vi "Set Live img window UI from file-DBL.vi"(8 "error in (no error)":errorcluster, 9 "Keys setup.DBL":T2, 10 "Section name":string, 11 "Refnum in":T1) -> (0 "error out":errorcluster, 3 "Refnum out":T1)   [LabVIEW 2020]
uses:
  Typedefs/Ini file interface (DBL).ctl
  <vilib>/Utility/config.llb/Config Data RefNum.ctl
  User Interface/Globals/gl_Windows Ctrl refs.vi
  <vilib>/Utility/config.llb/NI_LVConfig.lvlib
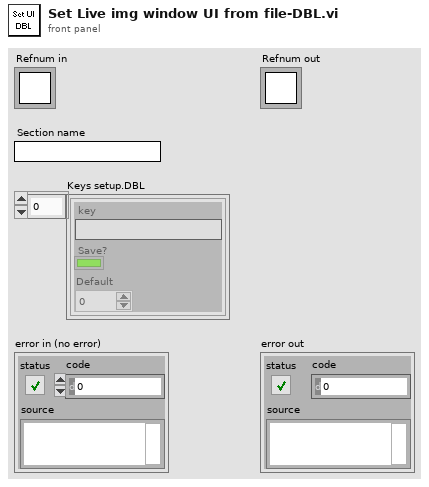
[diagram p1: front panel]
types:
  T1 = typedef "NI_LVConfig.lvlib/Config Data RefNum.ctl" = refnum<k1>
  T2 = typedef "Ini file interface (DBL).ctl" = cluster{"key":string, "Save?":bool, "Default":dbl}[]
  T3 = typedef "Live window-ctrl refs.ctl" = cluster{"This VI":refnum<vi>, "Pane":refnum<vi>, "Show REF Image Left":refnum<vi>, "Show REF Image Right":refnum<vi>, "Snapshot":refnum<vi>, "Left Image Palette":refnum<vi>, "Right Image Palette":refnum<vi>, "Left Channel":refnum<vi>, "Right Channel":refnum<vi>, "Left image intensity":refnum<vi>, "Right image intensity":refnum<vi>, "Left Image Display":T4, "Right Image Display":T4, "Refresh rate ind (Hz)":refnum<vi>, "Acq rate ind (Hz)":refnum<vi>, "Stop (ind)":refnum<vi>}
  T4 = typedef "Image display ref.ctl" = refnum<vi>
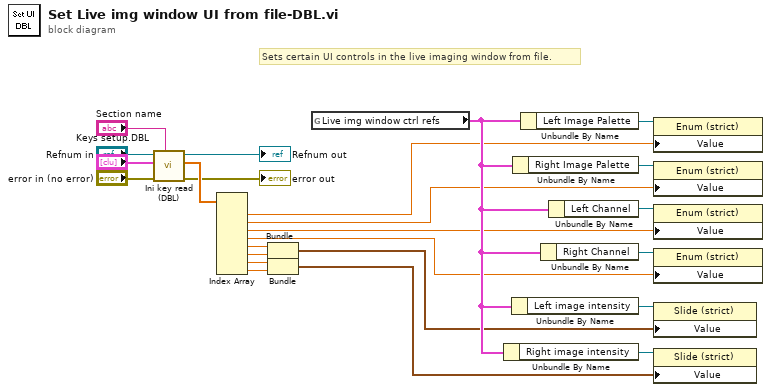
[diagram p0: block diagram]
diagram:
  # "Sets certain UI controls in the live imaging window from file."
  n1 = call "Ini key read (DBL).vi"("Section name"="Section name", "error in (no error)"="error in (no error)", "Parameter names & setup"="Keys setup.DBL", "Ini file refnum in"="Refnum in") -> ("error out"=→"error out":errorcluster, "Value read/used"=w22:dbl[], "Ini file refnum out"=→"Refnum out":T1)  [unwired: 5 in]
  n2 = Index Array(array=w22) -> (element #1=w10:dbl, element #2=w9:dbl, element #3=w8:dbl, element #4=w7:dbl, element #5=w6:dbl, element #6=w5:dbl, element #7=w3:dbl, element #8=w2:dbl)  [unwired: 8 in]
  n3 = Bundle("value"=w6, "value"=w5) -> (w4:cluster{"value":dbl, "value":dbl})  [unwired: 1 in]
  n4 = Bundle("value"=w3, "value"=w2) -> (w1:cluster{"value":dbl, "value":dbl})  [unwired: 1 in]
  n5 = global read "gl_Windows Ctrl refs.vi" "Live img window ctrl refs"() -> (w11:T3)
  n6 = Unbundle By Name(w11) -> ("Right image intensity"=w13:refnum<vi>)
  n7 = Unbundle By Name(w11) -> ("Left image intensity"=w12:refnum<vi>)
  n8 = Unbundle By Name(w11) -> ("Right Image Palette"=w16:refnum<vi>)
  n9 = Unbundle By Name(w11) -> ("Left Image Palette"=w17:refnum<vi>)
  n10 = Unbundle By Name(w11) -> ("Right Channel"=w15:refnum<vi>)
  n11 = Unbundle By Name(w11) -> ("Left Channel"=w14:refnum<vi>)
  n12 = property class="Enum (strict)"(reference=w17, "Value"=w10) -> ()  [unwired: 1 in, 2 out]
  n13 = property class="Enum (strict)"(reference=w16, "Value"=w9) -> ()  [unwired: 1 in, 2 out]
  n14 = property class="Enum (strict)"(reference=w14, "Value"=w8) -> ()  [unwired: 1 in, 2 out]
  n15 = property class="Enum (strict)"(reference=w15, "Value"=w7) -> ()  [unwired: 1 in, 2 out]
  n16 = property class="Slide (strict)"(reference=w12, "Value"=w4) -> ()  [unwired: 1 in, 2 out]
  n17 = property class="Slide (strict)"(reference=w13, "Value"=w1) -> ()  [unwired: 1 in, 2 out]
